vi "remove_waveforms.vi"(8 "error in (no error)":errorcluster, 11 "HSDIO in":refnum<class "HSDIO.lvclass">) -> (0 "error out":errorcluster, 3 "HSDIO out":refnum<class "HSDIO.lvclass">)   [LabVIEW 2013, in "HSDIO.lvclass"]
uses:
  HSDIO.lvclass
  HSDIO.lvclass/HSDIO.ctl
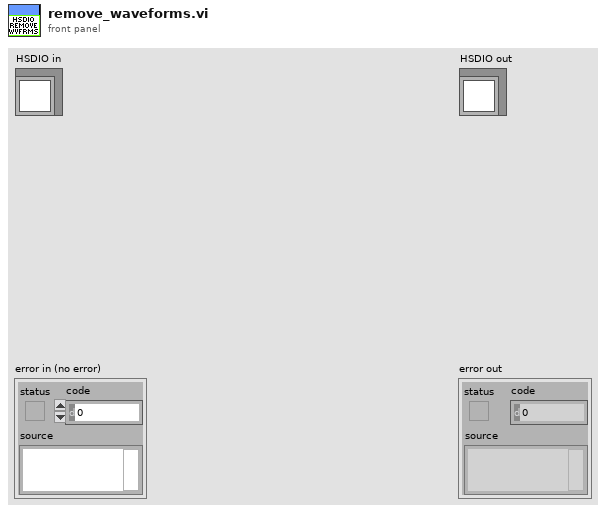
[diagram p1: front panel]
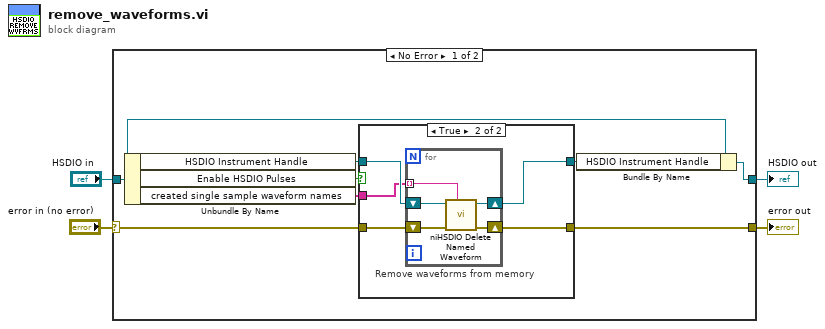
[diagram p0: block diagram]
diagram:
  n1 = case shown="No Error" "error in (no error)" {
    selector: "error in (no error)" -> [w11 w26]
    tunnel: [w6 w26] -> w3
    tunnel: [w9 w25] -> w1
    tunnel: "HSDIO in" -> [w10 w25]
    frame No Error {
      n2 = Unbundle By Name(w10) -> ("HSDIO Instrument Handle"=w12:refnum<k15>, "Enable HSDIO Pulses"=w7:bool, "created single sample waveform names"=w5:string[])
      n3 = case shown="True" w7 {
        tunnel: w12 -> [w13 w19]
        tunnel: [w13 w18] -> w8
        tunnel: w5 -> [_ w17]
        tunnel: w11 -> [w14 w16]
        tunnel: [w14 w15] -> w6
        frame False {
        }
        frame True {
          n4 = for "Remove waveforms from memory" {
            shift-right: [w20] -> w15
            shift-left: w16 -> [w21]
            shift-right: [w23] -> w18
            shift-left: w19 -> [w24]
            tunnel: w17 -> [w22] mode=indexing
            n5 = call <instrlib>:"niHSDIO Delete Named Waveform.vi"("waveform name (default:\"\")"=w22, "error in (no error)"=w21, "instrument handle"=w24) -> ("error out"=w20:errorcluster, "instrument handle out"=w23:refnum<k15>)  [unwired: 7 in]
          }
        }
      }
      n6 = Bundle By Name(cluster=w10, "HSDIO Instrument Handle"=w8) -> (w9:refnum<class "HSDIO.lvclass">)
    }
    frame Error {
    }
  }
  "error out" <- w3
  "HSDIO out" <- w1
